vi "CRISTALIZADOR_GLOBALES.vi"() -> ()   [LabVIEW 2017]
uses:
  CRISTALIZADOR_COMM.ctl
  AGILENT 34970/34970_Configuracion.ctl
  CRISTALIZADOR_parametrosMedida.ctl
  CRISTALIZADOR_datosEnsayo.ctl
panel:
  in  "datosEnsayo":T1 {"CAUDALIMETRO_HZ" format="%.2f"; "AGIT_TEMPERATURA_C" format="%.2f"; "AMB_TEMPERATURA_C" format="%.2f"; "TOUT_TEMPERATURA_C" format="%.2f"; "TIN_TEMPERATURA_C" format="%.2f"; "AGIT_PAR_NM" format="%.2f"; "AGIT_VELOCIDAD_RPM" format="%.2f"; "AGIT_SETPOINT_RPM" format="%.2f"; "T2_TEMPERATURA_C" format="%.2f"; "T1_TEMPERATURA_C" format="%.2f"; "TIEMPO_MIN" format="%.2f"}
  in  "Ensayo":T2={"Nombre ensayo"="Nombre ensayo", "Muestra"="Nombre fluido", "Promedios"=10, "Frecuencia adq(s)"=1.0, "Tiempo medida(min) "=10.0, "Tiempo ensayo(h) "=10.0} {"Frecuencia adq(s)" format="%.3f"}
  out "Dispositivos":T3=[["Temperatura", "PT100.1", "201", "C", "0.00"], ["Temperatura", "PT100.2", "202", "C", "0.00"], ["Temperatura", "PT100.3", "205", "C", "0.00"], ["Temperatura", "PT100.4", "210", "C", "0.00"], ["Temperatura", "Termopar K", "208", "C", "0.00"]] caption="configuracionCanales"
  in  "Comments":string
  in  "Stop_rotador":bool
  out "Sampling(s)":dbl format="%.1f"
  out "Comunicaciones":T4={"IKA_Eurostar"="ASRL6::INSTR", "IKA"=FALSE, "Agilent"="ASRL6::INSTR", "AGL"=FALSE, "SLOT AGL"=TRUE, "CAUDAL"=TRUE}
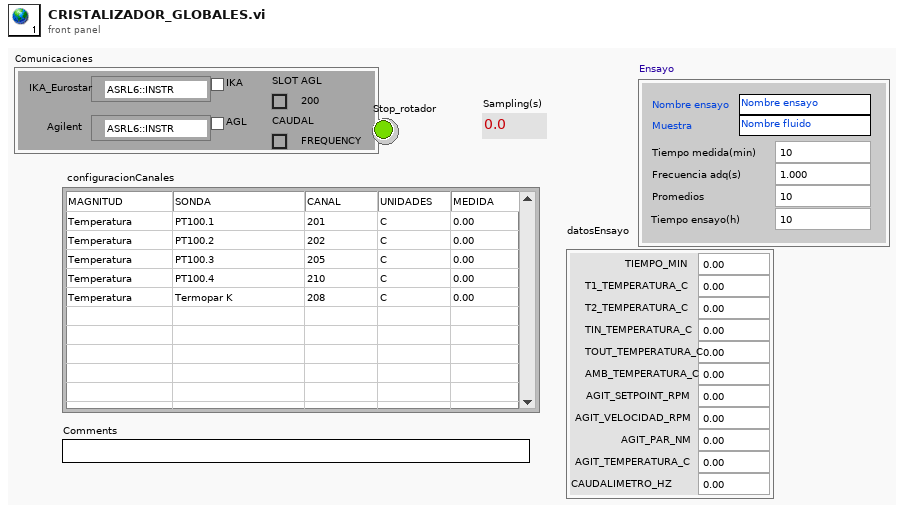
[diagram p1: front panel]
types:
  T1 = typedef "CRISTALIZADOR_datosEnsayo.ctl" = cluster{"TIEMPO_MIN":dbl, "T1_TEMPERATURA_C":dbl, "T2_TEMPERATURA_C":dbl, "TIN_TEMPERATURA_C":dbl, "TOUT_TEMPERATURA_C":dbl, "AMB_TEMPERATURA_C":dbl, "AGIT_SETPOINT_RPM":dbl, "AGIT_VELOCIDAD_RPM":dbl, "AGIT_PAR_NM":dbl, "AGIT_TEMPERATURA_C":dbl, "CAUDALIMETRO_HZ":dbl}
  T2 = typedef "CRISTALIZADOR_parametrosMedida.ctl" = cluster{"Nombre ensayo":string, "Muestra":string, "Promedios":u16, "Frecuencia adq(s)":dbl, "Tiempo medida(min) ":dbl, "Tiempo ensayo(h) ":dbl}
  T3 = typedef "34970_Configuracion.ctl" = string[][]
  T4 = typedef "CRISTALIZADOR_COMM.ctl" = cluster{"IKA_Eurostar":refnum<visa-resource-name>, "IKA":bool, "Agilent":refnum<visa-resource-name>, "AGL":bool, "SLOT AGL":bool, "CAUDAL":bool}
diagram:
